vi "Write outputs.vi"(5 "outputs":refnum<class "Terminal.lvclass">[](array[class]), 9 "Node in":refnum<class "Node.lvclass">) -> (3 "Node out":refnum<class "Node.lvclass">)   [LabVIEW 2014, in "Raspberry Pi Compatible Compiler for LabVIEW.lvlib" / "Node.lvclass"]
uses:
  Node.lvclass
  Terminal/Terminal.lvclass
  Node.lvclass/Node.ctl
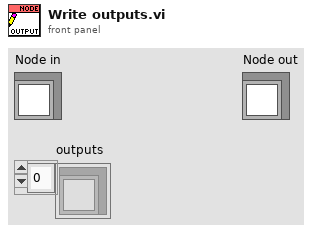
[diagram p1: front panel]
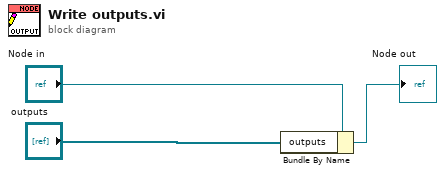
[diagram p0: block diagram]
diagram:
  n1 = Bundle By Name(cluster="Node in", "outputs"="outputs") -> (→"Node out":refnum<class "Node.lvclass">)
